vi "Dictionary to Map.vi"(8 "error in (no error)":errorcluster, 11 "Data (Dictionary)":T2[](array[typedef])) -> (0 "error out":errorcluster, 3 "map out":T1)   [LabVIEW 2019, in "LV-Data.lvclass"]
uses:
  LV-Data.lvclass
  Typedefs/Dictionary--cluster.ctl
  Typedefs/Map Variant--map.ctl
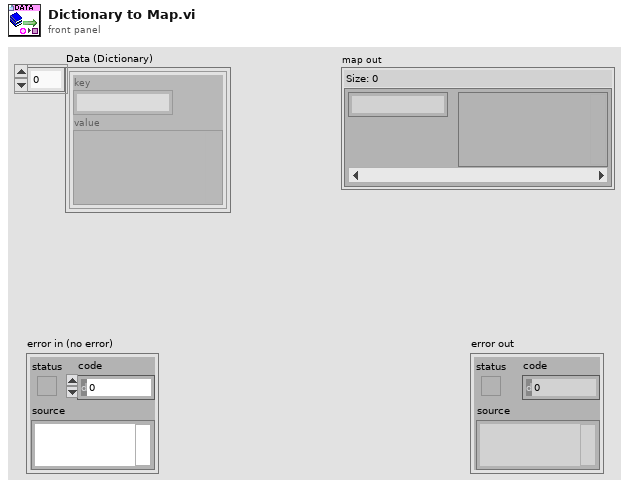
[diagram p1: front panel]
types:
  T1 = typedef "LV-Data.lvclass/Map Variant--map.ctl" = map{string, variant}
  T2 = typedef "LV-Data.lvclass/Dictionary--cluster.ctl" = cluster{"key":string, "value":variant}
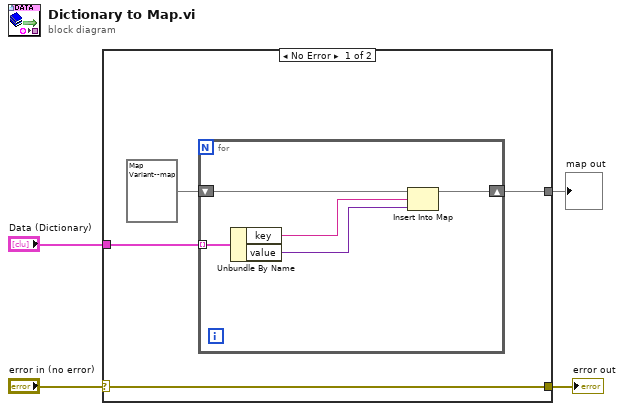
[diagram p0: block diagram]
diagram:
  n1 = case shown="No Error" "error in (no error)" {
    selector: "error in (no error)" -> [w8 w14]
    tunnel: [w8 w14] -> w3
    tunnel: "Data (Dictionary)" -> [w7 _]
    tunnel: [w6 _] -> w1
    frame No Error {
      n2 = for {
        tunnel: w7 -> [w13] mode=indexing
        shift-right: [w11] -> w6
        shift-left: T1 {} ("map in") -> [w9]
        n3 = Unbundle By Name(w13) -> ("key"=w12:string, "value"=w10:variant)
        n4 = Insert Into Map(map in=w9, key=w12, value=w10) -> (map out=w11:T1)  [unwired: 2 out]
      }
    }
    frame Error {
    }
  }
  "error out" <- w3
  "map out" <- w1
